vi "Create Data Channels.vi"(8 "error in":errorcluster, 11 "Node in":refnum<class "BLS Power Supply Template.lvclass">) -> (0 "error out":errorcluster, 3 "Node out":refnum<class "BLS Power Supply Template.lvclass">)   [LabVIEW 2023, in "BLS Power Supply Template.lvlib" / "BLS Power Supply Template.lvclass"]
uses:
  BLS Power Supply Template.lvclass
  C:/Program Files/National Instruments/LabVIEW 2023/vi.lib/ADAS Replay HIL/Template Node/Plugin/Template Node/Template Node.lvclass
  BLS Power Supply Template.lvclass/BLS Power Supply Template.ctl
  <vilib>/ADAS Replay HIL/Channels/Tag Wrapper/Polymorphic/Open Producer Tag (Double).vi
  <vilib>/ADAS Replay HIL/Channels/Tag Wrapper/Polymorphic/Open Producer Tag (Double).vi/45cd6eaa-a1ce-41a4-8aba-62a49d103d7e.vi
  <vilib>/ADAS Replay HIL/Channels/Tag Wrapper/Polymorphic/Open Producer Tag (Double).vi/45cd6eaa-a1ce-41a4-8aba-62a49d103d7e.vi/c28b0ead-42ad-4072-80a2-aca7f2bd7ce3.vi
  <vilib>/ADAS Replay HIL/Template Node/Plugin/Template Node/Data Channel/Get Tag Producer Channel Name.vi
  <vilib>/ADAS Replay HIL/AdasHilServices/AdasHilServices Fill In Error Info Ex.vi
  <vilib>/ADAS Replay HIL/Channels/Tag Wrapper/Tag Wrapper.lvlib
  <vilib>/ADAS Replay HIL/Template Node/Plugin/Template Node/Template Node.lvclass
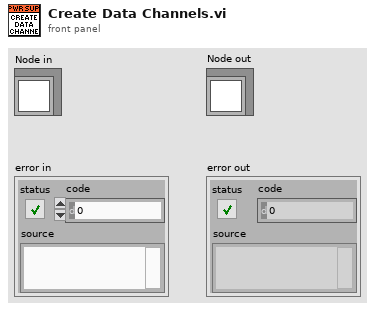
[diagram p1: front panel]
types:
  T1 = typedef "Template Node.lvlib/Template Node.lvclass/Data Channel Info.ctl" = cluster{"Channel Name":string, "Type Description":string}
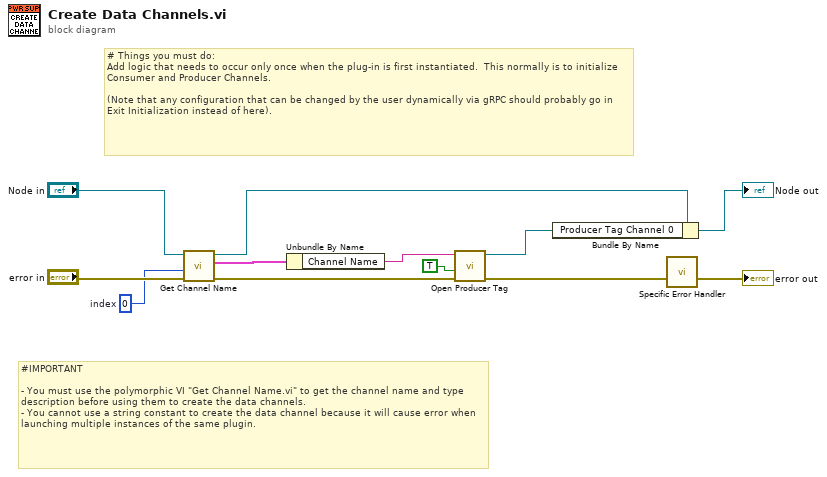
[diagram p0: block diagram]
diagram:
  w8 = 0  # index
  # "# Things you must do:\nAdd logic that needs to occur only once when the plug-in is first instantiated.  This normally is to initialize Consumer and Producer Channels.   \n\n(Note that any configuration that can be changed by the user dynamically via gRPC should probably go in Exit Initialization instead of here)."
  # "#IMPORTANT\n\n- You must use the polymorphic VI \"Get Channel Name.vi\" to get the channel name and type description before using them to create the data channels.\n- You cannot use a string constant to create the data channel because it will cause error when launching multiple instances of the same plugin."
  n1 = call-poly <vilib>:"Get Channel Name.vi"("error in"="error in", "index"=w8, "Node in"="Node in") -> ("error out"=w4:errorcluster, "Channel Name"=w7:T1, "Node out"=w9:refnum<class "BLS Power Supply Template.lvclass">)  [unwired: 6 in]
  n2 = Unbundle By Name(w7) -> ("Channel Name"=w5:string)
  n3 = call-poly <vilib>:"Open Producer Tag.vi"("error in"=w4, "Create if not found? (T)"=TRUE, "Channel Name"=w5) -> ("error out"=w3:errorcluster, "ADAS HIL Channel"=w2:refnum<k21>)  [unwired: 7 in]
  n4 = Bundle By Name(cluster=w9, "Producer Tag Channel 0"=w2) -> (→"Node out":refnum<class "BLS Power Supply Template.lvclass">)
  n5 = call "Specific Error Handler"("Error to Check"=w3) -> ("error out"=→"error out":errorcluster)  [unwired: 11 in, 3 out]
